vi "Update path and value.vi"(8 "error in (no error)":errorcluster, 10 "OME_MD_GUI control references":T1, 11 "Row Index":i32) -> (0 "error out":errorcluster)   [LabVIEW 2012]
doc: "SciScan 1.2 160622"
uses:
  Custom Controls and Typedefs/OME_MD_GUI control references.ctl
  Custom Controls and Typedefs/Objective Parameters Cluster.ctl
  Custom Controls and Typedefs/Experiment and Experimenter.ctl
  Custom Controls and Typedefs/Channel Parameters Cluster.ctl
panel:
  # "Experiment"
  # "Experimenter"
  # "Sample"
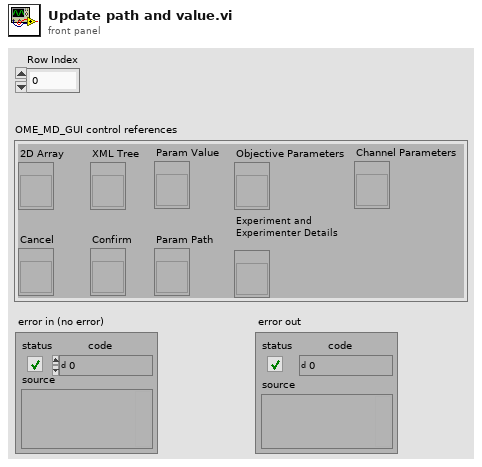
[diagram p1: front panel]
types:
  T1 = typedef "OME_MD_GUI control references.ctl" = cluster{"2D Array":refnum<vi>, "XML Tree":refnum<vi>, "Param Value":refnum<vi>, "Cancel":refnum<vi>, "Confirm":refnum<vi>, "Param Path":refnum<vi>, "Objective Parameters":refnum<vi>, "Experiment and Experimenter Details":refnum<vi>, "Channel Parameters":refnum<vi>}
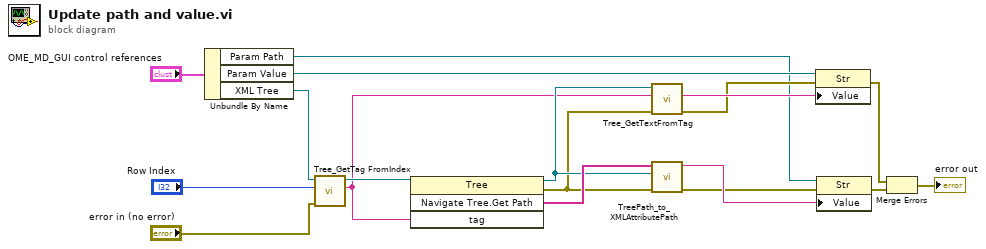
[diagram p0: block diagram]
diagram:
  n1 = Unbundle By Name("OME_MD_GUI control references") -> ("Param Path"=w3:refnum<vi>, "Param Value"=w4:refnum<vi>, "XML Tree"=w17:refnum<vi>)
  n2 = call "Tree_GetTag FromIndex.vi"("Error In"="error in (no error)", "Index IN"="Row Index", "Tree Refnum IN"=w17) -> ("Tag OUT"=w2:string, "Tree Refnum OUT"=w5:refnum<vi>)  [unwired: 6 in, 1 out]
  n3 = invoke class="Tree" method="Navigate Tree.Get Path"(reference=w5, "tag"=w2) -> (reference out=w12:refnum<vi>, error out=w10:errorcluster, "Navigate Tree:Get Path"=w13:string[])  [unwired: 2 in, 1 out]
  n4 = call "Tree_GetTextFromTag.vi"("Error In"=w10, "Tag IN"=w2, "Tree Refnum IN"=w12) -> ("Error Out"=w8:errorcluster, "String OUT"=w14:string)  [unwired: 6 in, 1 out]
  n5 = call "TreePath_to_XMLAttributePath.vi"("error in (no error)"=w10, "Tree Refnum"=w12, "Tree Path (Array)"=w13) -> ("error out"=w9:errorcluster, "XML Attribute path (String)"=w11:string)  [unwired: 6 in, 1 out]
  n6 = property class="Str"(reference=w4, error in=w8, "Value"=w14) -> (error out=w7:errorcluster)  [unwired: 1 out]
  n7 = property class="Str"(reference=w3, error in=w9, "Value"=w11) -> (error out=w6:errorcluster)  [unwired: 1 out]
  n8 = Merge Errors(w7, w6) -> (→"error out":errorcluster)
